vi "Get Tuner Gain.vi"(8 "error in (no error)":errorcluster, 11 "DeviceRefnum":u64) -> (0 "error out":errorcluster, 2 "Gain (dB)":dbl, 3 "DeviceRefnum Out":u64)   [LabVIEW 2014]
doc: "RTLSDR_API int rtlsdr_get_tuner_gain(rtlsdr_dev_t *dev);"
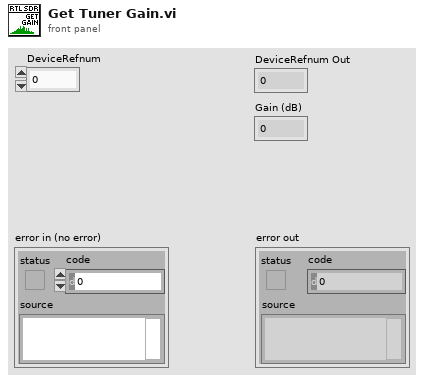
[diagram p1: front panel]
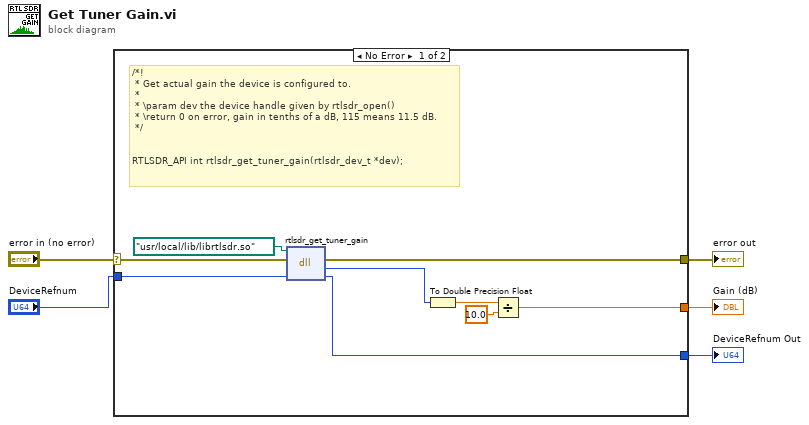
[diagram p0: block diagram]
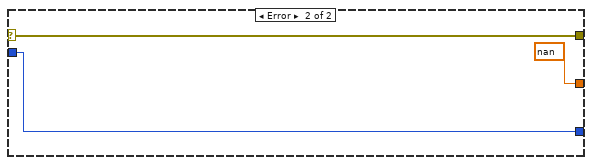
[diagram p2: hidden frame]
diagram:
  n1 = case shown="No Error" "error in (no error)" {
    selector: "error in (no error)" -> [w7 w17]
    tunnel: [w14 w17] -> w5
    tunnel: [w11 nan] -> w4
    tunnel: "DeviceRefnum" -> [w10 w16]
    tunnel: [w9 w16] -> w2
    frame No Error {
      # "/*!\n * Get actual gain the device is configured to.\n *\n * \\param dev the device handle given by rtlsdr_open()\n * \\return 0 on error, gain in tenths of a dB, 115 means 11.5 dB.\n */\n\n\nRTLSDR_API int rtlsdr_get_tuner_gain(rtlsdr_dev_t *dev);"
      n2 = dll-call lib="C:/Program Files (x86)/National Instruments/LabVIEW 2016/user.lib/rtlsdr/rtlsdr.*" fn="rtlsdr_get_tuner_gain"(path in=path "/usr/local/lib/librtlsdr.so", error in=w7, "DeviceRefnum"=w10) -> (error out=w14:errorcluster, "Gain"=w6:i32, "DeviceRefnum"=w9:u64)  [unwired: 1 in, 1 out]
      n3 = To Double Precision Float(number=w6) -> (double precision float=w13:dbl)
      n4 = Divide(x=w13, y=10.0) -> (x/y=w11:dbl)
    }
    frame Error {
    }
  }
  "error out" <- w5
  "Gain (dB)" <- w4
  "DeviceRefnum Out" <- w2
